vi "networkstreamWrite.vi"(4 "Array":cluster{"x":dbl, "y":dbl}[](array[cluster])) -> ()   [LabVIEW 2014]
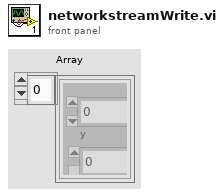
[diagram p1: front panel]
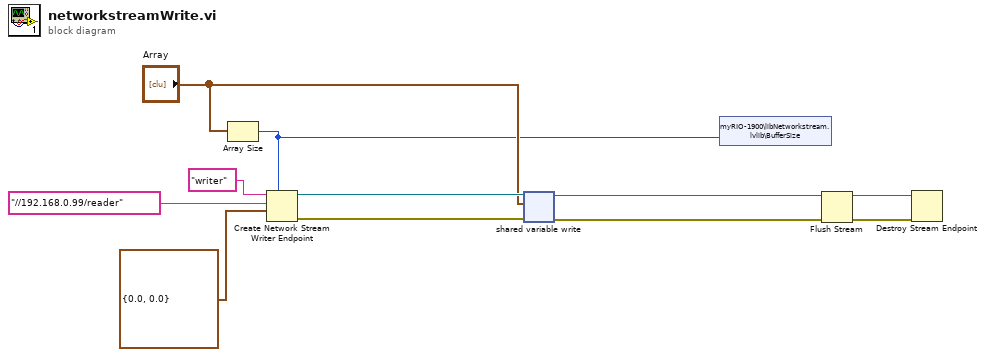
[diagram p0: block diagram]
diagram:
  n1 = Array Size(array="Array") -> (size(s)=w1:i32)
  n2 = Create Network Stream Writer Endpoint(7:w1, 9:cluster{dbl, dbl} {0.0, 0.0}, 10:"//192.168.0.99/reader" ("reader url"), 11:"writer" ("writer name")) -> (0:w4:errorcluster, 3:w3:refnum<k21>)  [unwired: 3 in]
  n3 = shared-variable-write(w3, w4, "Array") -> (w8:refnum<k21>, w9:errorcluster)  [unwired: 1 in, 1 out]
  n4 = shared-variable "myRIO-1900\\libNetworkstream.lvlib\\BufferSize"(w1) -> ()  [unwired: 1 in, 1 out]
  n5 = Flush Stream(8:w9, 11:w8) -> (0:w10:errorcluster, 3:w11:refnum<k21>)  [unwired: 2 in, 1 out]
  n6 = Destroy Stream Endpoint(8:w10, 11:w11) -> ()  [unwired: 1 out]
